vi "Set X Voltage.vi"(8 "error in (no error)":errorcluster, 10 "Set x Voltage(V)":dbl, 11 "hdl in":i32) -> (0 "error out":errorcluster, 3 "hdl":i32)   [LabVIEW 2011, in "Thorlabs_MDT69xB.lvlib"]
doc: "Set the output voltage for the X axis."
uses:
  <instrlib>/Thorlabs_MDT69xB/Thorlabs_MDT69xB.lvlib
  <instrlib>/Thorlabs_MDT69xB/Data/MDT_COMMAND_LIB_win32.dll
  <instrlib>/Thorlabs_MDT69xB/Data/MDT_COMMAND_LIB_x64.dll
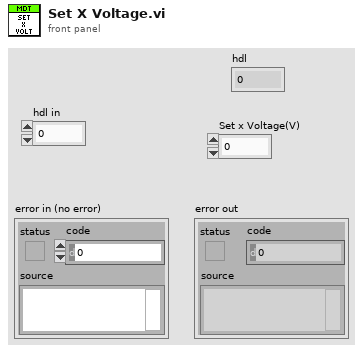
[diagram p1: front panel]
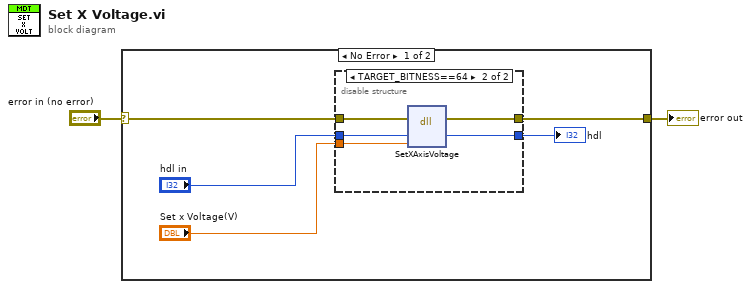
[diagram p0: block diagram]
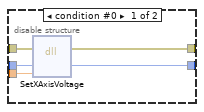
[diagram p2: hidden frame]
diagram:
  n1 = case shown="No Error" "error in (no error)" {
    selector: "error in (no error)" -> [w7 w18]
    tunnel: [w4 w18] -> w1
    frame No Error {
      n2 = disable-structure shown="TARGET_BITNESS==64" {
        disable-tunnel: w7 -> [w12 w17]
        disable-tunnel: "hdl in" -> [w11 w16]
        disable-tunnel: "Set x Voltage(V)" -> [w10 w15]
        disable-tunnel: [w9 w14] -> w4
        disable-tunnel: [w8 w13] -> w3
        frame condition #0 {
          n3 = dll-call lib="C:/Program Files (x86)/National Instruments/LabVIEW 2011/instr.lib/Thorlabs_MDT69xB/Data/MDT_COMMAND_LIB_win32.dll" fn="SetXAxisVoltage"(error in=w12, "hdl"=w11, "voltage"=w10) -> (error out=w9:errorcluster, "hdl"=w8:i32)  [unwired: 4 in, 1 out]
        }
        frame condition #1 (active) {
          n4 = dll-call lib="C:/Program Files/National Instruments/LabVIEW 2011/instr.lib/Thorlabs_MDT69xB/Data/MDT_COMMAND_LIB_x64.dll" fn="SetXAxisVoltage"(error in=w17, "hdl"=w16, "voltage"=w15) -> (error out=w14:errorcluster, "hdl"=w13:i32)  [unwired: 4 in, 1 out]
        }
      }
      "hdl" <- w3
    }
    frame Error {
    }
  }
  "error out" <- w1
